vi "json.generate_object.vi"(8 "error in":errorcluster, 11 "timestampMetadata in":refnum<class "timestampMetadata.lvclass">) -> (0 "error out":errorcluster, 2 "JSON Object":string, 3 "timestampMetadata out":refnum<class "timestampMetadata.lvclass">)   [LabVIEW 2018, in "timestampMetadata.lvclass"]
uses:
  timestampMetadata.lvclass
  timestampMetadata.lvclass/timestampMetadata.ctl
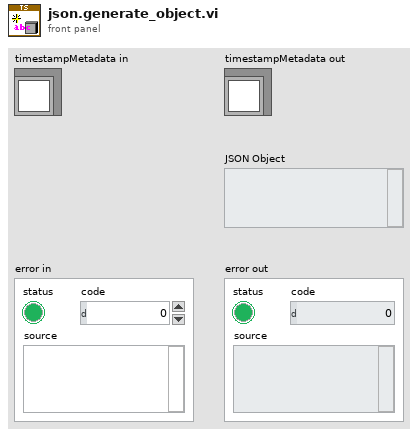
[diagram p1: front panel]
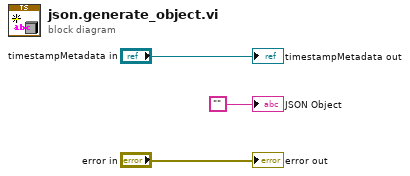
[diagram p0: block diagram]
diagram:
  "timestampMetadata out" <- "timestampMetadata in"
  "error out" <- "error in"
  "JSON Object" <- ""
